vi "CRYWrite Range.vi"(1 "In Items":string[](array[string]), 2 "In Unit":string) -> ()   [LabVIEW 2013]
uses:
  CRYMainGlobal.vi
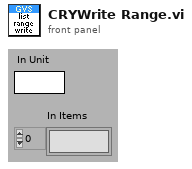
[diagram p1: front panel]
types:
  T1 = enum16{"open", "replace", "create", "open or create", "replace or create", "replace or create with confirmation"}
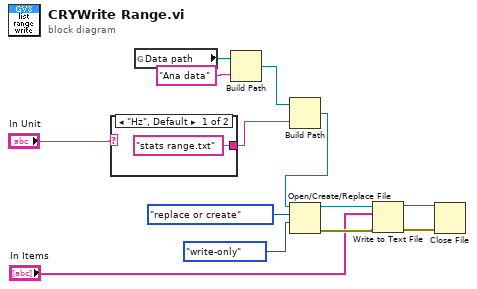
[diagram p0: block diagram]
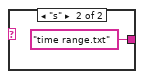
[diagram p2: hidden frame]
diagram:
  n1 = case shown="\"Hz\", Default" "In Unit" {
    tunnel: ["stats range.txt" ("name or relative path") "time range.txt" ("name or relative path")] -> w8
    frame "Hz", Default {
    }
    frame "s" {
    }
  }
  n2 = global read "CRYMainGlobal.vi" "Data path"() -> (w1:path)
  n3 = Build Path(base path=w1, name or relative path="Ana data") -> (appended path=w2:path)
  n4 = Build Path(base path=w2, name or relative path=w8) -> (appended path=w7:path)
  n5 = Open/Create/Replace File(file path (use dialog)=w7, operation (0:open)=T1."replace or create", access (0:read/write)=enum16{"read/write", "read-only", "write-only"}."write-only") -> (refnum out=w11:refnum<file>, error out=w12:errorcluster)  [unwired: 1 in, 3 out]
  n6 = Write to Text File(file (use dialog)=w11, text="In Items", error in=w12) -> (refnum out=w13:refnum<file>, error out=w4:errorcluster)  [unwired: 2 out]
  n7 = Close File(refnum=w13, error in=w4) -> ()  [unwired: 2 out]
